vi "CTRE_CANifier_SetPWMOutput.vi"(8 "error in":errorcluster, 9 "PWMChannel":T1, 10 "Duty Cycle":dbl min=0.0 max=1.0 step=0.01 format="%#_13g", 11 "CANifierDevRef":T2) -> (0 "error out":errorcluster, 3 "CANifierDevRef":T2)   [LabVIEW 2019]
uses:
  <vilib>/Rock Robotics/WPI/ThirdParty/Phoenix-LabVIEW/CANifier/CTRE_CANifier_DeviceRef.ctl
  <vilib>/Rock Robotics/WPI/ThirdParty/Phoenix-LabVIEW/CANifier/CTRE_CANifier_PWMChannel.ctl
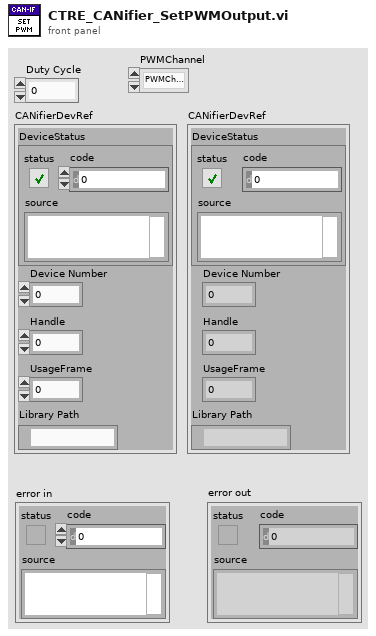
[diagram p1: front panel]
types:
  T1 = typedef "CTRE_CANifier_PWMChannel.ctl" = enum16{"PWMChannel0", "PWMChannel1", "PWMChannel2", "PWMChannel3"}
  T2 = typedef "CTRE_CANifier_DeviceRef.ctl" = cluster{"DeviceStatus":errorcluster, "Device Number":u8, "Handle":u64, "UsageFrame":u32, "Library Path":path}
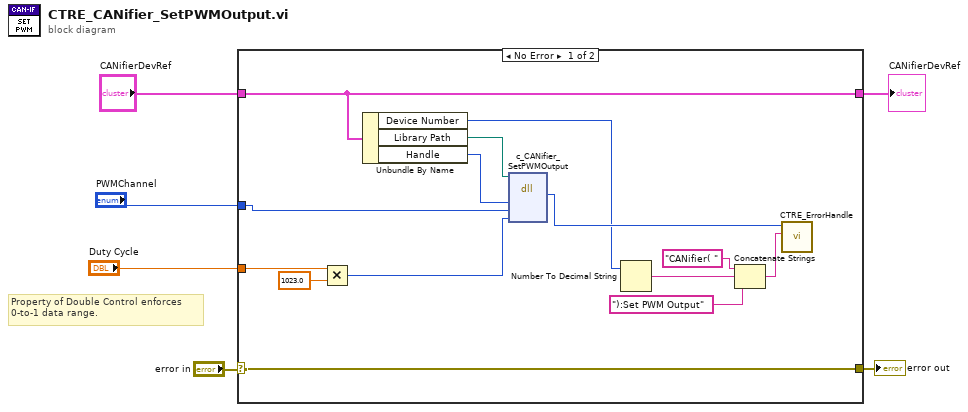
[diagram p0: block diagram]
diagram:
  # "Property of Double Control enforces\n0-to-1 data range."
  n1 = case shown="No Error" "error in" {
    selector: "error in" -> [w20 w22]
    tunnel: [w20 w22] -> w5
    tunnel: "PWMChannel" -> [w8 _]
    tunnel: "Duty Cycle" -> [w19 _]
    tunnel: "CANifierDevRef" -> [w17 w21]
    tunnel: [w17 w21] -> w2
    frame No Error {
      n2 = Multiply(x=w19, y=1023.0) -> (x*y=w7:u32)
      n3 = Unbundle By Name(w17) -> ("Device Number"=w10:u8, "Library Path"=w16:path, "Handle"=w15:u64)
      n4 = dll-call lib="?" fn="c_CANifier_SetPWMOutput"(path in=w16, "handle"=w15, "pwmChannel"=w8, "dutyCycle"=w7) -> ("CTR_Code"=w14:i8)  [unwired: 5 in, 2 out]
      n5 = Number To Decimal String(number=w10) -> (decimal integer string=w13:string)  [unwired: 1 in]
      n6 = Concatenate Strings("CANifier( " ("string"), w13, "):Set PWM Output" ("string")) -> (w9:string)
      n7 = call <vilib>:"CTRE_ErrorHandle.vi"("origin"=w9, "code"=w14) -> ()  [unwired: 9 in, 1 out]
    }
    frame Error {
    }
  }
  "error out" <- w5
  "CANifierDevRef" <- w2
